vi "Initialize_Keithley.vi"(8 "error in (no error)":errorcluster, 10 "Parameter":T1={"Ch1 MeasRange"="2E-6", "Ch2 MeasRange"="2E-6", "Ch1 SourceRange"="10", "Ch2 SourceRange"="10", "Ch1 SourceOutput"="0", "Ch2 SourceOutput"="0"}, 11 "VISA resource name":refnum<visa-resource-name>) -> (0 "error out":errorcluster, 3 "VISA resource name out":refnum<visa-resource-name>)   [LabVIEW 2013]
doc: "Input (Example)\n-------------------\nMeasRange (2E-6)\nSourceRange (10)\nSourceOutput (0)"
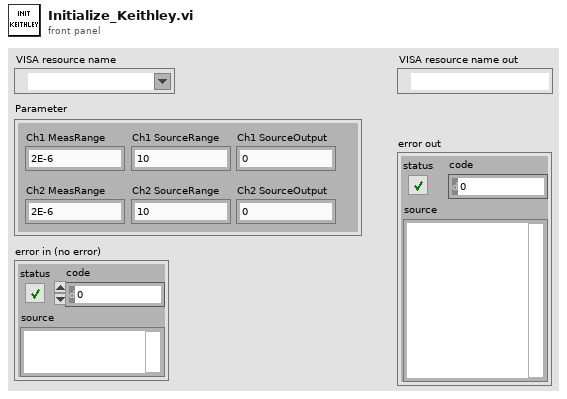
[diagram p1: front panel]
types:
  T1 = cluster{"Ch1 MeasRange":string, "Ch2 MeasRange":string, "Ch1 SourceRange":string, "Ch2 SourceRange":string, "Ch1 SourceOutput":string, "Ch2 SourceOutput":string}
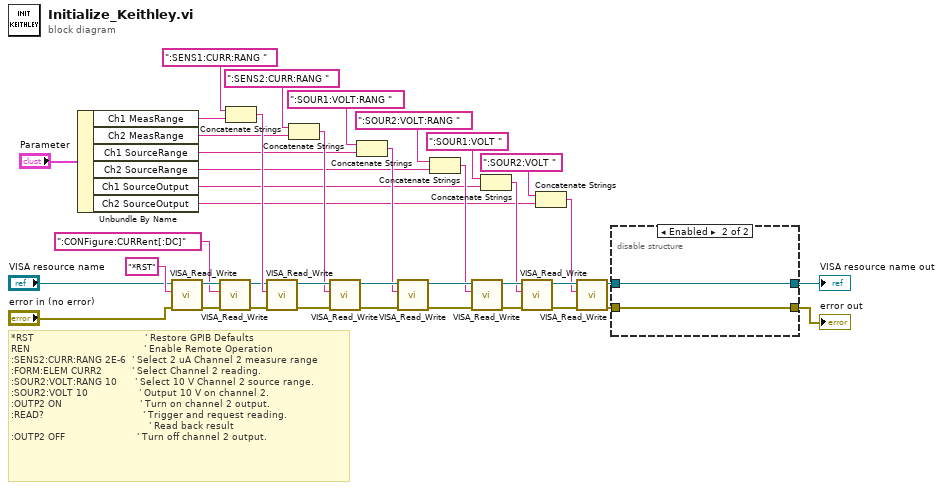
[diagram p0: block diagram]
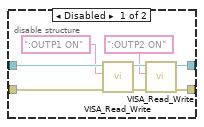
[diagram p2: hidden frame]
diagram:
  # "*RST \t\t\t                                 ' Restore GPIB Defaults\nREN                                      ' Enable Remote Operation\n:SENS2:CURR:RANG 2E-6 \t' Select 2 uA Channel 2 measure range\n:FORM:ELEM CURR2 \t        ' Select Channel 2 reading.\n:SOUR2:VOLT:RANG 10 \t    ' Select 10 V Channel 2 source range.\n:SOUR2:VOLT 10 \t\t              ' Output 10 V on channel 2.\n:OUTP2 ON \t\t                       ' Turn on channel 2 output.\n:READ? \t\t\t                             ' Trigger and request reading.\n\t\t\t                                           ' Read back result\n:OUTP2 OFF \t\t                     ' Turn off channel 2 output."
  n1 = Unbundle By Name("Parameter") -> ("Ch1 MeasRange"=w16:string, "Ch2 MeasRange"=w14:string, "Ch1 SourceRange"=w12:string, "Ch2 SourceRange"=w10:string, "Ch1 SourceOutput"=w9:string, "Ch2 SourceOutput"=w7:string)
  n2 = call "VISA_Read_Write.vi"("error in (no error)"="error in (no error)", "write buffer"="*RST", "VISA resource name"="VISA resource name") -> ("error out"=w5:errorcluster, "VISA resource name out"=w4:refnum<visa-resource-name>)  [unwired: 5 in, 2 out]
  n3 = call "VISA_Read_Write.vi"("error in (no error)"=w5, "write buffer"=":CONFigure:CURRent[:DC]", "VISA resource name"=w4) -> ("error out"=w2:errorcluster, "VISA resource name out"=w3:refnum<visa-resource-name>)  [unwired: 5 in, 2 out]
  n4 = Concatenate Strings(":SENS1:CURR:RANG ", w16) -> (w17:string)
  n5 = call "VISA_Read_Write.vi"("error in (no error)"=w2, "write buffer"=w17, "VISA resource name"=w3) -> ("error out"=w38:errorcluster, "VISA resource name out"=w37:refnum<visa-resource-name>)  [unwired: 5 in, 2 out]
  n6 = Concatenate Strings(":SENS2:CURR:RANG ", w14) -> (w15:string)
  n7 = call "VISA_Read_Write.vi"("error in (no error)"=w38, "write buffer"=w15, "VISA resource name"=w37) -> ("error out"=w35:errorcluster, "VISA resource name out"=w36:refnum<visa-resource-name>)  [unwired: 5 in, 2 out]
  n8 = Concatenate Strings(":SOUR1:VOLT:RANG ", w12) -> (w13:string)
  n9 = call "VISA_Read_Write.vi"("error in (no error)"=w35, "write buffer"=w13, "VISA resource name"=w36) -> ("error out"=w33:errorcluster, "VISA resource name out"=w34:refnum<visa-resource-name>)  [unwired: 5 in, 2 out]
  n10 = Concatenate Strings(":SOUR2:VOLT:RANG ", w10) -> (w11:string)
  n11 = call "VISA_Read_Write.vi"("error in (no error)"=w33, "write buffer"=w11, "VISA resource name"=w34) -> ("error out"=w32:errorcluster, "VISA resource name out"=w31:refnum<visa-resource-name>)  [unwired: 5 in, 2 out]
  n12 = Concatenate Strings(":SOUR1:VOLT ", w9) -> (w8:string)
  n13 = call "VISA_Read_Write.vi"("error in (no error)"=w32, "write buffer"=w8, "VISA resource name"=w31) -> ("error out"=w29:errorcluster, "VISA resource name out"=w30:refnum<visa-resource-name>)  [unwired: 5 in, 2 out]
  n14 = Concatenate Strings(":SOUR2:VOLT ", w7) -> (w6:string)
  n15 = call "VISA_Read_Write.vi"("error in (no error)"=w29, "write buffer"=w6, "VISA resource name"=w30) -> ("error out"=w27:errorcluster, "VISA resource name out"=w28:refnum<visa-resource-name>)  [unwired: 5 in, 2 out]
  n16 = disable-structure shown="Enabled" {
    disable-tunnel: w28 -> [w49 w51]
    disable-tunnel: w27 -> [w48 w50]
    disable-tunnel: [w43 w51] -> w26
    disable-tunnel: [w42 w50] -> w25
    frame Disabled {
      n17 = call "VISA_Read_Write.vi"("error in (no error)"=w48, "write buffer"=":OUTP1 ON", "VISA resource name"=w49) -> ("error out"=w46:errorcluster, "VISA resource name out"=w47:refnum<visa-resource-name>)  [unwired: 5 in, 2 out]
      n18 = call "VISA_Read_Write.vi"("error in (no error)"=w46, "write buffer"=":OUTP2 ON", "VISA resource name"=w47) -> ("error out"=w42:errorcluster, "VISA resource name out"=w43:refnum<visa-resource-name>)  [unwired: 5 in, 2 out]
    }
    frame Enabled {
    }
  }
  "VISA resource name out" <- w26
  "error out" <- w25
